vi "integral.vi"(10 "Starting value":dbl, 11 "x":dbl) -> (3 "Integral x":dbl)   [LabVIEW 2015]
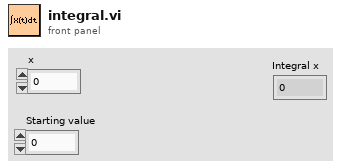
[diagram p1: front panel]
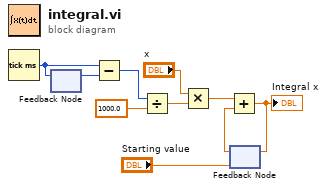
[diagram p0: block diagram]
diagram:
  n1 = Tick Count (ms)() -> (millisecond timer value=w8:u32)
  n2 = feedback #1() -> (w9:u32)  [unwired: 1 in]
  n3 = feedback-in #1(w8) -> ()
  n4 = Subtract(x=w8, y=w9) -> (x-y=w3:u32)
  n5 = Divide(x=w3, y=1000.0) -> (x/y=w1:dbl)
  n6 = Multiply(x="x", y=w1) -> (x*y=w6:dbl)
  n7 = feedback #2("Starting value") -> (w4:dbl)
  n8 = Add(x=w6, y=w4) -> (x+y=w5:dbl)
  "Integral x" <- w5
  n9 = feedback-in #2(w5) -> ()
